vi "about read notes section.vi"(7 "Parent Path (empty)":path, 8 "error in (no error)":errorcluster, 10 "Section Name (\"\")":string, 11 "refnum":T2) -> (0 "error out":errorcluster, 1 "Submodules":T1(array[cluster]), 2 "Date":string, 3 "dup refnum":T2, 4 "Notes":string[](array[string]), 5 "Version":string, 6 "Models":string[](array[string]))   [LabVIEW 2011]
uses:
  <vilib>/Utility/config.llb/Config Data RefNum.ctl
  <vilib>/Utility/config.llb/Read Key (String).vi
  <vilib>/Utility/config.llb/NI_LVConfig.lvlib
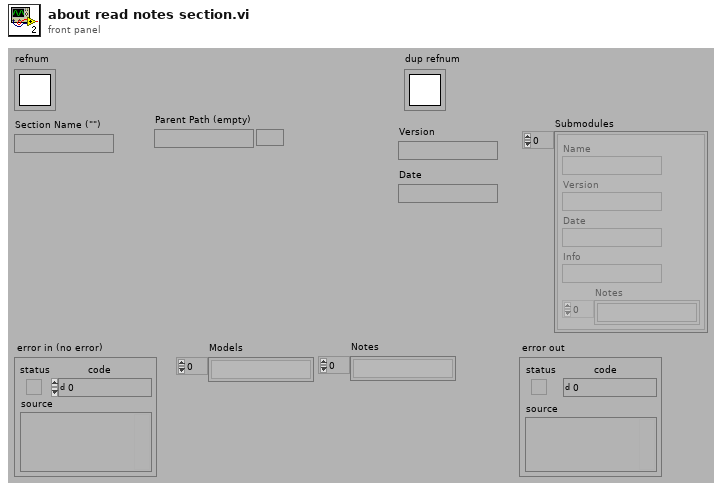
[diagram p1: front panel]
types:
  T1 = cluster{"Name":string, "Version":string, "Date":string, "Info":string, "Notes":string[]}[]
  T2 = typedef "NI_LVConfig.lvlib/Config Data RefNum.ctl" = refnum<k1>
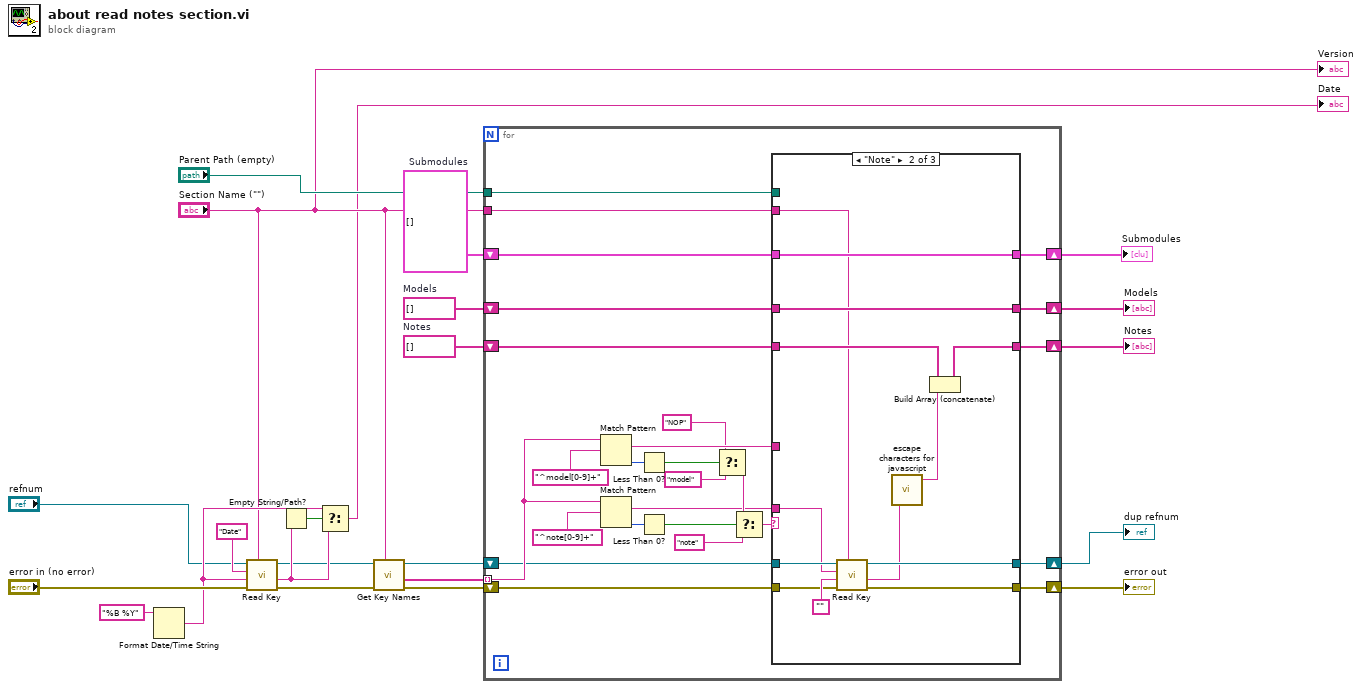
[diagram p0: block diagram]
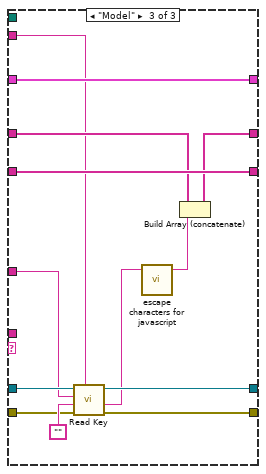
[diagram p3: hidden frame]
diagram:
  w12 = T1 []  # Submodules
  w16 = string[] []  # Models
  w18 = string[] []  # Notes
  n1 = Format Date/Time String(time format string (%c)="%B %Y") -> (date/time string=w6:string)  [unwired: 2 out]
  n2 = call-poly <vilib>:"Read Key.vi"("section"="Section Name (\"\")", "error in (no error)"="error in (no error)", "default value"=w6, "key"="Date" ("Template (\"\")"), "refnum"="refnum") -> ("error out"=w1:errorcluster, "value"=w7:string, "refnum out"=w2:T2)  [unwired: 1 in, 3 out]
  n3 = Empty String/Path?(string/path=w7) -> (empty?=w9:bool)
  n4 = Select(t=w6, s=w9, f=w7) -> (s? t:f=→"Date":string)
  n5 = call <vilib>:"Get Key Names.vi"("section"="Section Name (\"\")", "error in (no error)"=w1, "refnum"=w2) -> ("error out"=w22:errorcluster, "key names"=w23:string[], "refnum out"=w21:T2)  [unwired: 6 out]
  n6 = for {
    shift-right: [w31] -> w17
    shift-left: w18 -> [w32]
    tunnel: w23 -> [w46] mode=indexing
    shift-right: [w33] -> w19
    shift-left: w21 -> [w34]
    shift-right: [w35] -> w20
    shift-left: w22 -> [w36]
    tunnel: "Section Name (\"\")" -> [w27]
    shift-right: [w29] -> w14
    shift-left: w16 -> [w30]
    tunnel: "Parent Path (empty)" -> [w28]
    shift-right: [w25] -> w13
    shift-left: w12 -> [w26]
    n7 = Match Pattern(string=w46, regular expression="^model[0-9]+") -> (match substring=w37:string, offset past match=w47:i32)  [unwired: 3 out]
    n8 = Match Pattern(string=w46, regular expression="^note[0-9]+") -> (match substring=w38:string, offset past match=w48:i32)  [unwired: 3 out]
    n9 = Less Than 0?(x=w47) -> (x < 0?=w42:bool)
    n10 = Less Than 0?(x=w48) -> (x < 0?=w44:bool)
    n11 = Select(t="NOP", s=w42, f="model") -> (s? t:f=w40:string)
    n12 = Select(t=w40, s=w44, f="note") -> (s? t:f=w39:string)
    n13 = case shown="\"Note\"" w39 {
      tunnel: w38 -> [_ w59 _]
      tunnel: w37 -> [_ _ w75]
      tunnel: [w54 w63 w76] -> w35
      tunnel: w36 -> [w54 w66 w79]
      tunnel: w34 -> [w53 w65 w78]
      tunnel: [w53 w64 w77] -> w33
      tunnel: w32 -> [w52 w62 w74]
      tunnel: [w52 w61 w74] -> w31
      tunnel: w30 -> [w51 w60 w73]
      tunnel: [w51 w60 w72] -> w29
      tunnel: w28 -> [_ _ _]
      tunnel: w27 -> [_ w57 w70]
      tunnel: w26 -> [w50 w58 w71]
      tunnel: [w50 w58 w71] -> w25
      frame "NOP", Default {
      }
      frame "Note" {
        n14 = call-poly <vilib>:"Read Key.vi"("section"=w57, "error in (no error)"=w66, "default value"="", "key"=w59, "refnum"=w65) -> ("error out"=w63:errorcluster, "value"=w56:string, "refnum out"=w64:T2)  [unwired: 1 in, 3 out]
        n15 = call "escape characters for javascript.vi"("String (\"\")"=w56) -> ("escaped String"=w55:string)  [unwired: 4 out]
        n16 = Build Array (concatenate)(w62, w55) -> (w61:string[])
      }
      frame "Model" {
        n17 = call-poly <vilib>:"Read Key.vi"("section"=w70, "error in (no error)"=w79, "default value"="", "key"=w75, "refnum"=w78) -> ("error out"=w76:errorcluster, "value"=w69:string, "refnum out"=w77:T2)  [unwired: 1 in, 3 out]
        n18 = call "escape characters for javascript.vi"("String (\"\")"=w69) -> ("escaped String"=w68:string)  [unwired: 4 out]
        n19 = Build Array (concatenate)(w73, w68) -> (w72:string[])
      }
    }
  }
  "error out" <- w20
  "dup refnum" <- w19
  "Notes" <- w17
  "Models" <- w14
  "Submodules" <- w13
  "Version" <- "Section Name (\"\")"
